vi "PositionNetTrainer.vi"() -> ()   [LabVIEW 2016]
panel:
  in  "Learning Rate":dbl
  in  "Stop Training":bool
  in  "Continue":bool
  in  "Start Training":bool
  out "Test Error":dbl[](graph)
  out "Training Error":dbl[](graph)
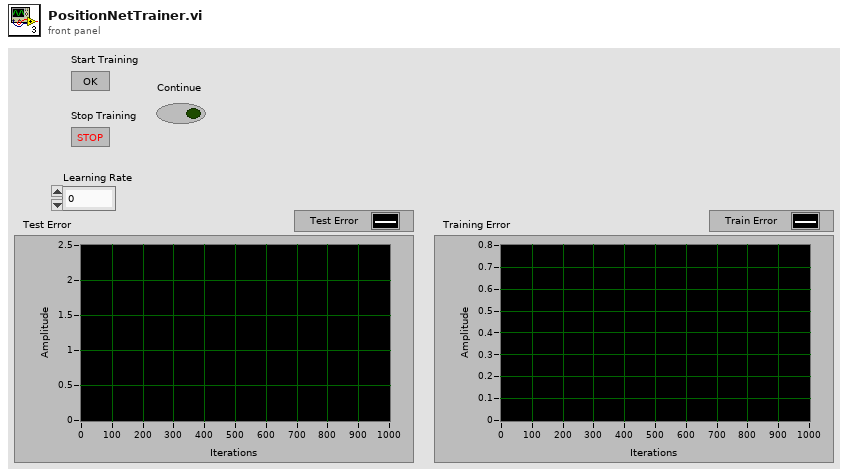
[diagram p1: front panel]
types:
  T1 = typedef "NI_Matrix.lvlib/RealMatrix.ctl" = dbl[][]
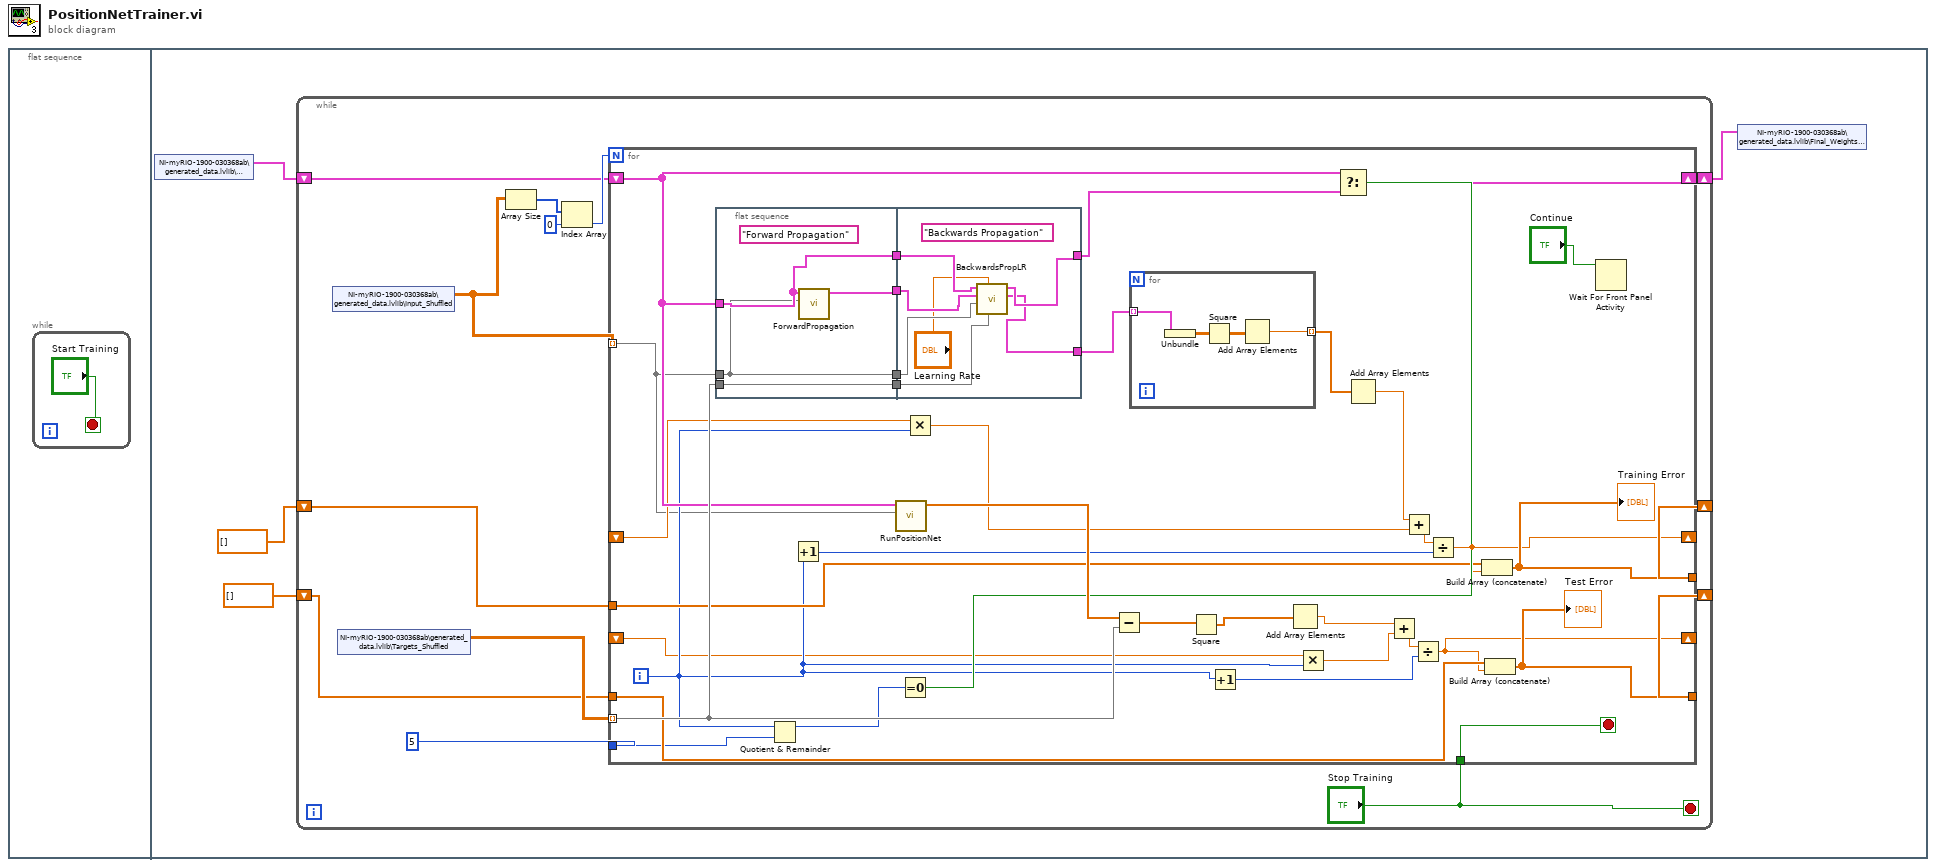
[diagram p0: block diagram]
diagram:
  n1 = flat-sequence {
    frame #0 {
      n2 = while {
        stop <- "Start Training" stop-if-true
      }
    }
    frame #1 {
      n3 = shared-variable "NI-myRIO-1900-030368ab\\generated_data.lvlib\\Weights_1"() -> (w5:cluster{dbl[][]}[])  [unwired: 1 in, 1 out]
      n4 = while {
        shift-right: [w14] -> w4
        shift-left: w5 -> [w15]
        shift-right: [w7] -> _
        shift-left: dbl[] [] -> [w9]
        shift-right: [w6] -> _
        shift-left: dbl[] [] -> [w8]
        stop <- "Stop Training" stop-if-true
        n5 = shared-variable "NI-myRIO-1900-030368ab\\generated_data.lvlib\\Input_Shuffled"() -> (w12:dbl[][])  [unwired: 1 in, 1 out]
        n6 = shared-variable "NI-myRIO-1900-030368ab\\generated_data.lvlib\\Targets_Shuffled"() -> (w18:dbl[][])  [unwired: 1 in, 1 out]
        n7 = Array Size(array=w12) -> (size(s)=w11:i32[])
        n8 = Index Array(array=w11, index=0) -> (element=w16:i32)
        n9 = for {
          N: w16 -> [_]
          tunnel: w12 -> [w20] mode=indexing
          tunnel: w18 -> [w48] mode=indexing
          shift-right: [w43] -> w14
          shift-left: w15 -> [w45]
          shift-right: [w33] -> _
          shift-left: _ -> [w36]
          shift-right: [w25] -> _
          shift-left: _ -> [w28]
          tunnel: 5 -> [w21]
          tunnel: "Stop Training" -> [w19]
          tunnel: w9 -> [w41]
          tunnel: [w42] -> w7
          tunnel: w8 -> [w40]
          tunnel: [w39] -> w6
          i -> [w29]
          stop <- w19 stop-if-true
          n10 = flat-sequence {
            tunnel: w45 -> [w61]
            tunnel: w20 -> [w60]
            tunnel: [w62] -> w54
            tunnel: w48 -> [w62]
            tunnel: [w59] -> w53
            tunnel: [w61] -> w52
            tunnel: [w60] -> w51
            tunnel: w54 -> [w67]
            tunnel: w53 -> [w65]
            tunnel: w52 -> [w64]
            tunnel: w51 -> [w66]
            tunnel: [w68] -> w50
            tunnel: [w69] -> w44
            frame #0 {
              (unwired) "Forward Propagation"
              n11 = call "ForwardPropagation.vi"("Input"=w60, "Weights"=w61) -> ("Y vectors"=w59:cluster{dbl[]}[])  [unwired: 9 in]
            }
            frame #1 {
              (unwired) "Backwards Propagation"
              n12 = call "BackwardsPropLR.vi"("Target"=w67, "Learning Rate"="Learning Rate", "Input"=w66, "Y vectors"=w65, "Weights"=w64) -> ("J"=w68:cluster{"Outer Product":T1}[], "Output Weights"=w69:cluster{"A - B":T1}[])  [unwired: 5 in]
            }
          }
          n13 = Quotient & Remainder(x=w29, y=w21) -> (x-y*floor(x/y)=w47:i32)  [unwired: 1 out]
          n14 = Increment(x=w29) -> (x+1=w32:i32)
          n15 = call "RunPositionNet.vi"("Input Vector"=w20, "Weights"=w45) -> ("Output Vector"=w49:dbl[])  [unwired: 9 in]
          n16 = Equal To 0?(x=w47) -> (x = 0?=w46:bool)
          n17 = Multiply(x=w36, y=w29) -> (x*y=w35:dbl)
          n18 = Subtract(x=w49, y=w48) -> (x-y=w38:dbl[])
          n19 = for {
            tunnel: w50 -> [w56] mode=indexing
            tunnel: [w55] -> w24 mode=indexing
            n20 = Unbundle(w56) -> ("Outer Product"=w58:T1)
            n21 = Square(x=w58) -> (x^2=w57:T1)
            n22 = Add Array Elements(numeric array=w57) -> (sum=w55:dbl)
          }
          n23 = Square(x=w38) -> (x^2=w37:dbl[])
          n24 = Increment(x=w29) -> (x+1=w30:i32)
          n25 = Add Array Elements(numeric array=w37) -> (sum=w26:dbl)
          n26 = Multiply(x=w28, y=w29) -> (x*y=w27:dbl)
          n27 = Select(t=w45, s=w46, f=w44) -> (s? t:f=w43:cluster{"A - B":T1}[])
          n28 = Add Array Elements(numeric array=w24) -> (sum=w23:dbl)
          n29 = Add(x=w26, y=w27) -> (x+y=w31:dbl)
          n30 = Add(x=w23, y=w35) -> (x+y=w34:dbl)
          n31 = Divide(x=w31, y=w30) -> (x/y=w25:dbl)
          n32 = Divide(x=w34, y=w32) -> (x/y=w33:dbl)
          n33 = Build Array (concatenate)(w41, w33) -> (w42:dbl[])
          "Training Error" <- w42
          n34 = Build Array (concatenate)(w40, w25) -> (w39:dbl[])
          "Test Error" <- w39
          n35 = Wait For Front Panel Activity(3:"Continue") -> ()  [unwired: 2 in, 1 out]
        }
      }
      n36 = shared-variable "NI-myRIO-1900-030368ab\\generated_data.lvlib\\Final_Weights_2"(w4) -> ()  [unwired: 1 in, 1 out]
    }
  }
